vi "Derive Send Method Path.vi"(8 "error in (no error)":errorcluster, 11 "Library":refnum<vi>) -> (0 "error out":errorcluster, 1 "found?":bool, 2 "Send VI Path":path)   [LabVIEW 2020, in "Message Rescripter.lvlib"]
uses:
  Message Rescripter.lvlib
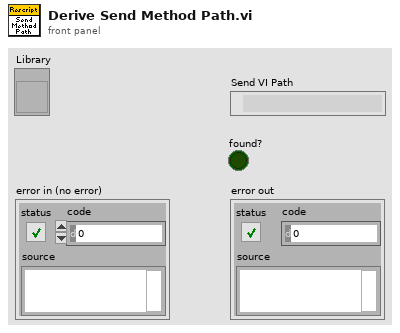
[diagram p1: front panel]
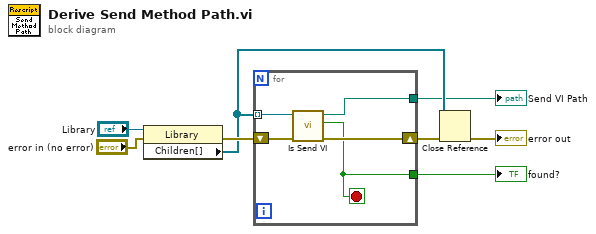
[diagram p0: block diagram]
diagram:
  n1 = property class="Library"(reference="Library", error in="error in (no error)") -> (error out=w8:errorcluster, "Children[]"=w7:refnum<vi>[])  [unwired: 1 out]
  n2 = for {
    tunnel: w7 -> [w12] mode=indexing
    shift-right: [w11] -> w6
    shift-left: w8 -> [w13]
    tunnel: [w9] -> w4
    tunnel: [w10] -> w3
    stop <- w10 stop-if-true
    n3 = call "Is Send VI.vi"("error in (no error)"=w13, "ProjectItem in"=w12) -> ("error out"=w11:errorcluster, "Is Send VI?"=w10:bool, "Path"=w9:path)  [unwired: 7 in]
  }
  "Send VI Path" <- w4
  "found?" <- w3
  n4 = Close Reference(reference=w7, error in (no error)=w6) -> (error out=→"error out":errorcluster)
